vi "example_relativeAlignment.vi"() -> ()   [LabVIEW 2023]
doc: "This example shows how to use the Relative Alignment VIs to align a 'movingObject' with an 'anchorObject'."
uses:
  <vilib>/numeric/Random Number (Range) U64.vi
  <vilib>/numeric/sub_Random U32.vi
panel:
  in  "alignHorizontalCenters":bool
  in  "alignVerticalCenters":bool
  in  "alignBottom":bool
  in  "alignTop":bool
  in  "useControlBodyOnly":bool=TRUE caption="Use Ctrl Body Only\n(=ignore labels \n& captions)"
  in  "stop":bool
  in  "alignRight":bool
  in  "alignLeft":bool
  in  "shuffle":bool
  in  "anchorObject":string
  in  "movingObject":dbl
  # "Instruction:\n1. Press Shuffle button to place the target objects randomly.\n2. Press the Alignment button you prefer."
  # "Relative alignment"
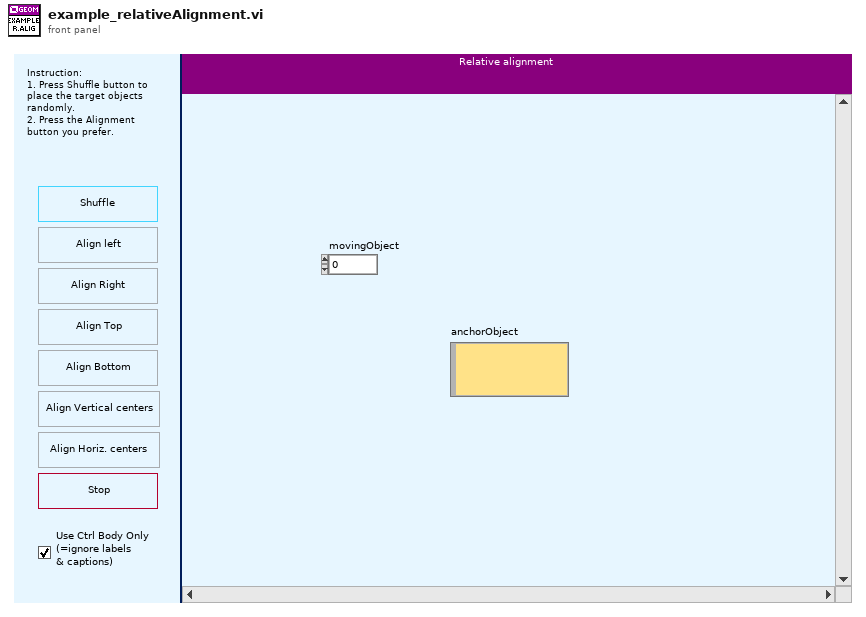
[diagram p1: front panel]
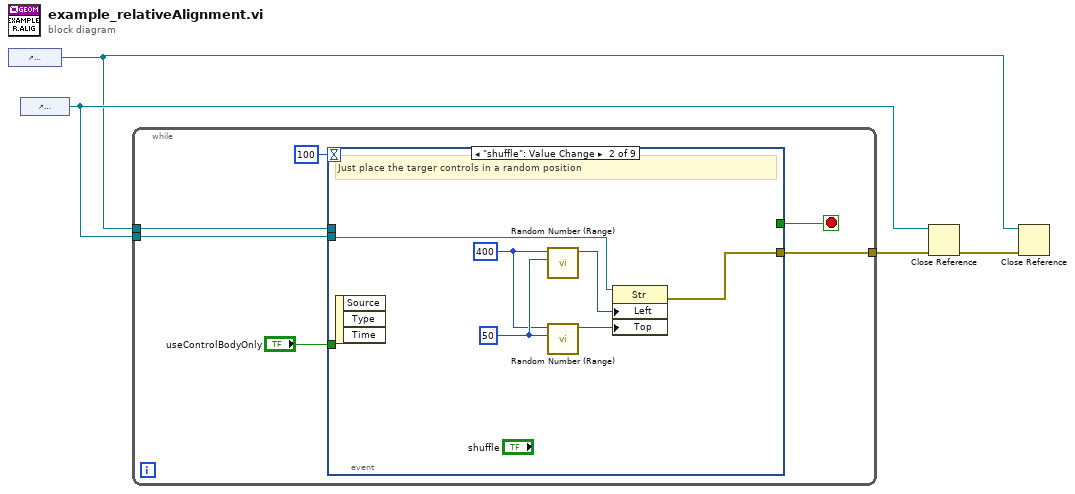
[diagram p0: block diagram]
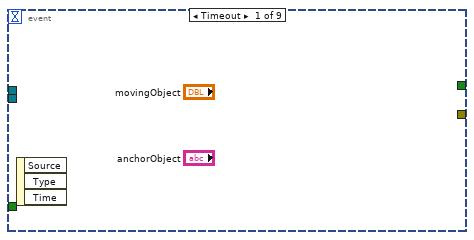
[diagram p2: hidden frame]
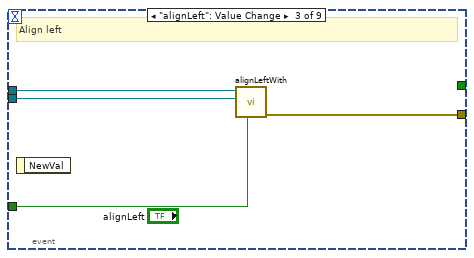
[diagram p3: hidden frame]
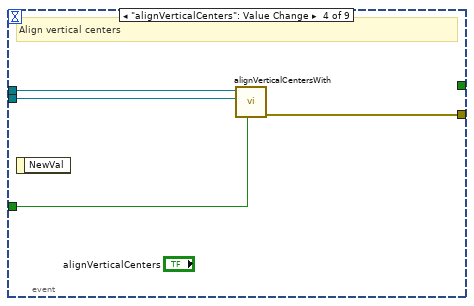
[diagram p4: hidden frame]
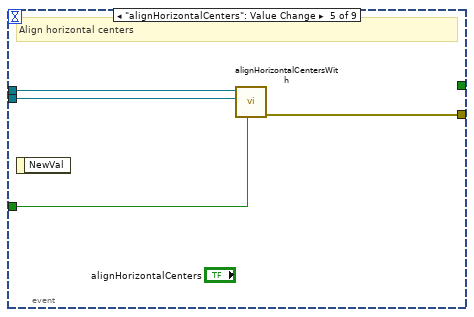
[diagram p5: hidden frame]
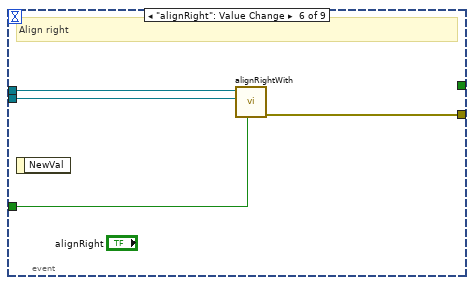
[diagram p6: hidden frame]
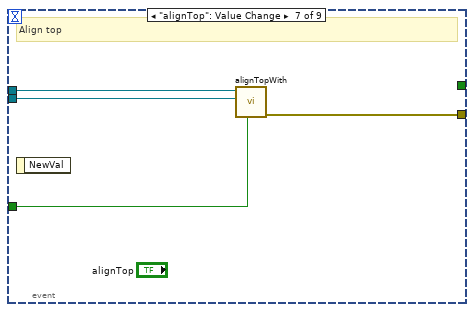
[diagram p7: hidden frame]
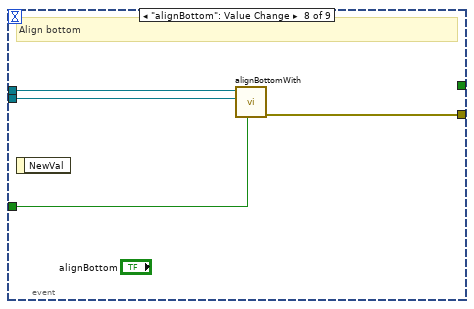
[diagram p8: hidden frame]
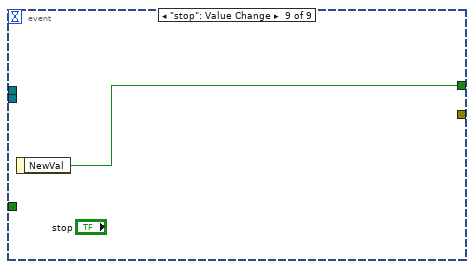
[diagram p9: hidden frame]
diagram:
  n1 = control-ref of="movingObject"() -> (w1:refnum<vi>)
  n2 = control-ref of="anchorObject"() -> (w2:refnum<vi>)
  n3 = while {
    tunnel: w2 -> [w9]
    tunnel: [w8] -> w4
    tunnel: w1 -> [w6]
    stop <- w10 stop-if-true
    n4 = event shown="[1] \"shuffle\": Value Change" {
      selector: _ -> [_ _ _ _ _ _ _ _ _]
      dyn-events: _ -> [_ _ _ _ _ _ _ _ _]
      timeout: 100 -> [_ _ _ _ _ _ _ _ _]
      tunnel: [_ _ _ _ _ _ _ _ w41] -> w10
      tunnel: w9 -> [_ w16 w18 w22 w26 w30 w34 w38 _]
      tunnel: [_ w15 w19 w23 w27 w31 w35 w39 _] -> w8
      tunnel: "useControlBodyOnly" -> [_ _ w20 w24 w28 w32 w36 w40 _]
      tunnel: w6 -> [_ _ w17 w21 w25 w29 w33 w37 _]
      event Timeout {
        n5 = event-data() -> ()  [unwired: 1 in, 3 out]
      }
      event "shuffle": Value Change {
        w11 = u64 400 ("lower bound (0)")
        w12 = u64 50 ("lower bound (0)")
        # "Just place the targer controls in a random position"
        n6 = event-data() -> ()  [unwired: 1 in, 3 out]
        n7 = call-poly <vilib>:"Random Number (Range).vi"("lower bound (0)"=w12, "upper bound (100)"=w11) -> ("number"=w14:u64)  [unwired: 9 in]
        n8 = call-poly <vilib>:"Random Number (Range).vi"("lower bound (0)"=w12, "upper bound (100)"=w11) -> ("number"=w13:u64)  [unwired: 9 in]
        n9 = property class="Str"(reference=w16, "Left"=w14, "Top"=w13) -> (error out=w15:errorcluster)  [unwired: 1 in, 1 out]
      }
      event "alignLeft": Value Change {
        # "Align left"
        n10 = event-data() -> ()  [unwired: 1 in, 1 out]
        n11 = call "alignLeftWith.vi"("useControlBodyOnly"=w20, "anchorObject"=w18, "movingObject"=w17) -> ("error out"=w19:errorcluster)  [unwired: 6 in, 2 out]
      }
      event "alignVerticalCenters": Value Change {
        # "Align vertical centers"
        n12 = event-data() -> ()  [unwired: 1 in, 1 out]
        n13 = call "alignVerticalCentersWith.vi"("useControlBodyOnly"=w24, "anchorObject"=w22, "movingObject"=w21) -> ("error out"=w23:errorcluster)  [unwired: 6 in, 2 out]
      }
      event "alignHorizontalCenters": Value Change {
        # "Align horizontal centers"
        n14 = event-data() -> ()  [unwired: 1 in, 1 out]
        n15 = call "alignHorizontalCentersWith.vi"("useControlBodyOnly"=w28, "anchorObject"=w26, "movingObject"=w25) -> ("error out"=w27:errorcluster)  [unwired: 6 in, 2 out]
      }
      event "alignRight": Value Change {
        # "Align right"
        n16 = event-data() -> ()  [unwired: 1 in, 1 out]
        n17 = call "alignRightWith.vi"("useControlBodyOnly"=w32, "anchorObject"=w30, "movingObject"=w29) -> ("error out"=w31:errorcluster)  [unwired: 6 in, 2 out]
      }
      event "alignTop": Value Change {
        # "Align top"
        n18 = event-data() -> ()  [unwired: 1 in, 1 out]
        n19 = call "alignTopWith.vi"("useControlBodyOnly"=w36, "anchorObject"=w34, "movingObject"=w33) -> ("error out"=w35:errorcluster)  [unwired: 6 in, 2 out]
      }
      event "alignBottom": Value Change {
        # "Align bottom"
        n20 = event-data() -> ()  [unwired: 1 in, 1 out]
        n21 = call "alignBottomWith.vi"("useControlBodyOnly"=w40, "anchorObject"=w38, "movingObject"=w37) -> ("error out"=w39:errorcluster)  [unwired: 6 in, 2 out]
      }
      event "stop": Value Change {
        n22 = event-data() -> ("NewVal"=w41:bool)  [unwired: 1 in]
      }
    }
  }
  n23 = Close Reference(reference=w2, error in (no error)=w4) -> (error out=w3:errorcluster)
  n24 = Close Reference(reference=w1, error in (no error)=w3) -> ()  [unwired: 1 out]
